vi "Rock Wall .vi"() -> ()   [LabVIEW 2015]
uses:
  AutoEnum.ctl
panel:
  in  "Encoder":dbl
  in  "Yaw":dbl
  in  "Ultrasonic":dbl
  in  "Distance Goal":dbl
  out "Rock Wall On":bool
  out "Motor Speed":dbl
  in  "Clear Error":bool
  in  "To Distance":bool
  out "Rest_Encoder":bool
  out "Rest_Gyro":bool
  in  "Enable":bool
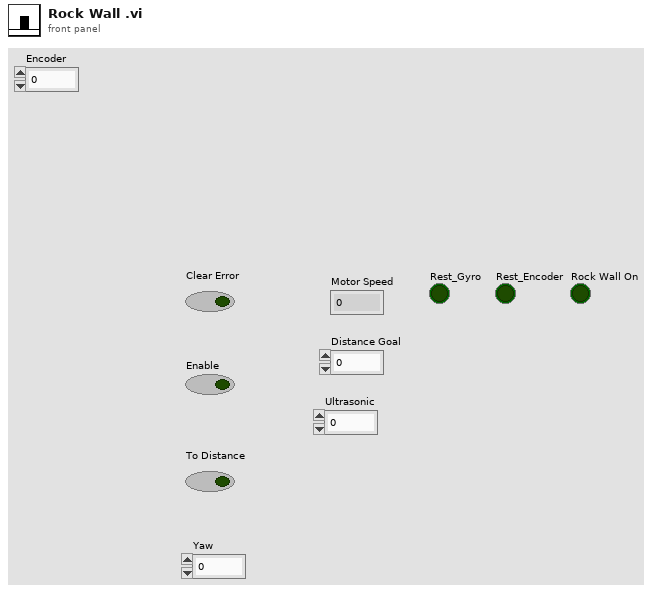
[diagram p1: front panel]
types:
  T1 = typedef "AutoEnum.ctl" = enum16{"Off", "ResetVar", "ResetOff", "BeforeTeeter", "LowerArm", "DriveForward", "Stop"}
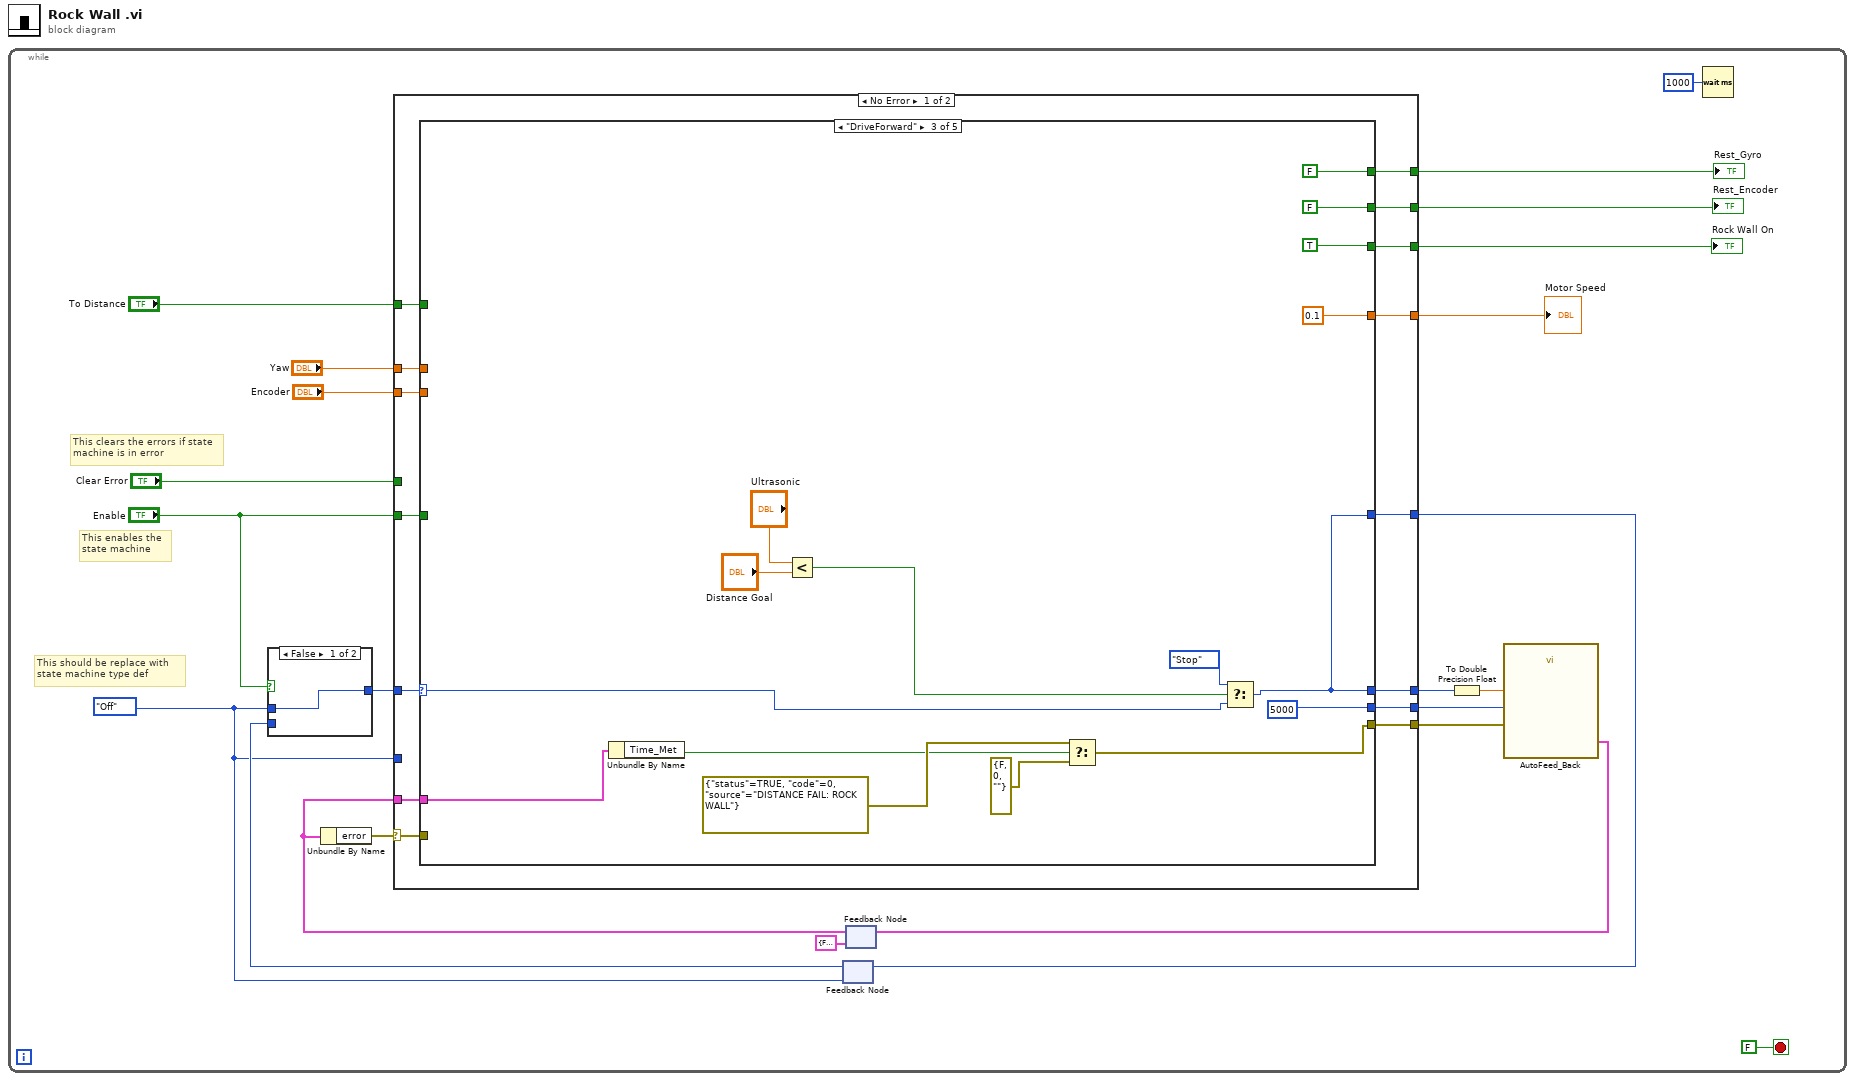
[diagram p0: block diagram]
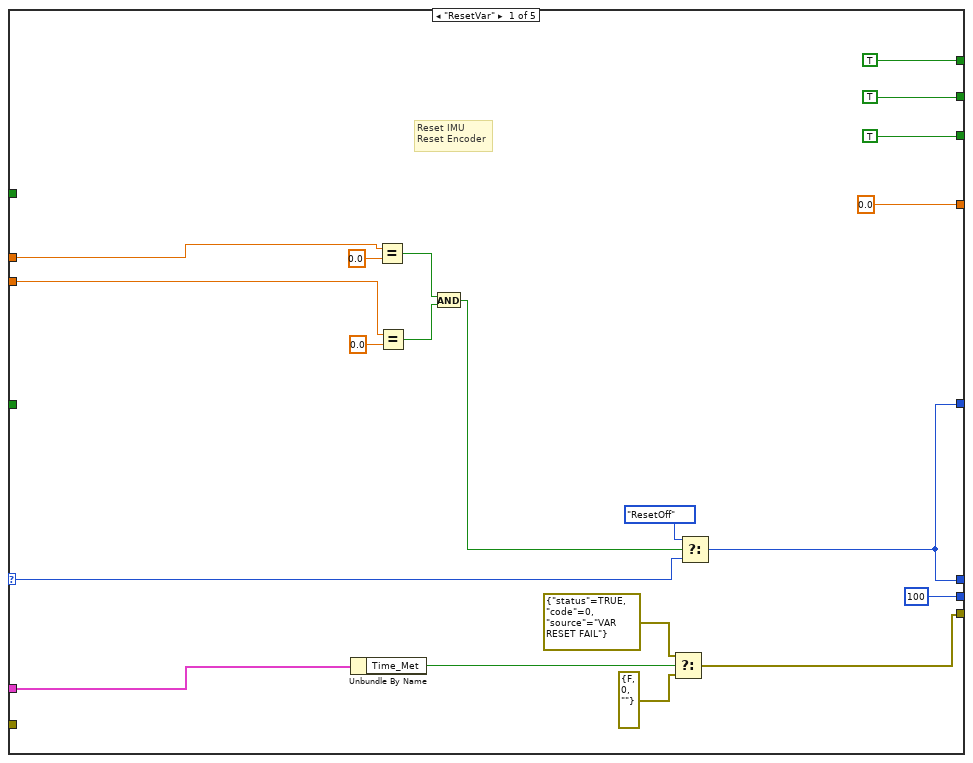
[diagram p3: hidden frame]
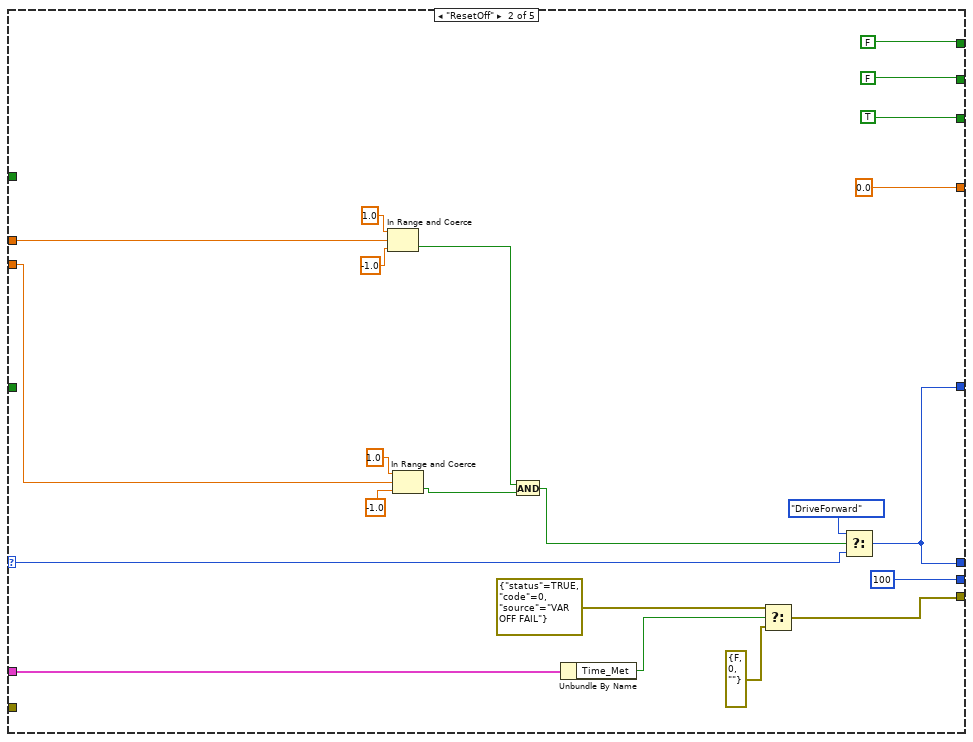
[diagram p4: hidden frame]
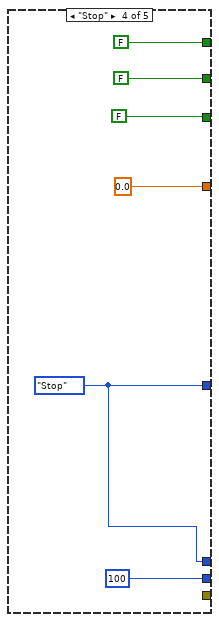
[diagram p5: hidden frame]
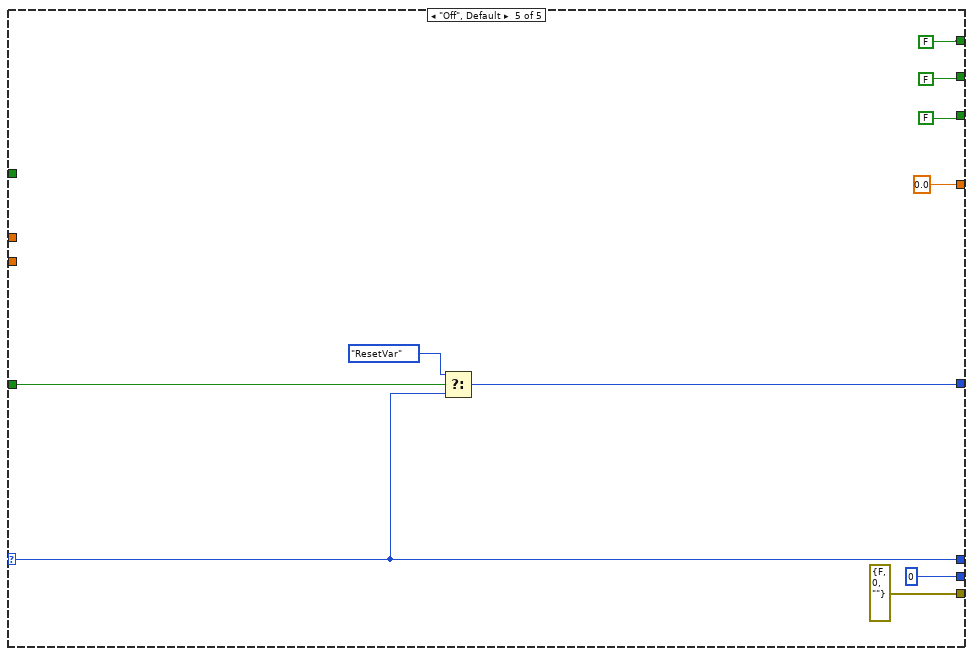
[diagram p6: hidden frame]
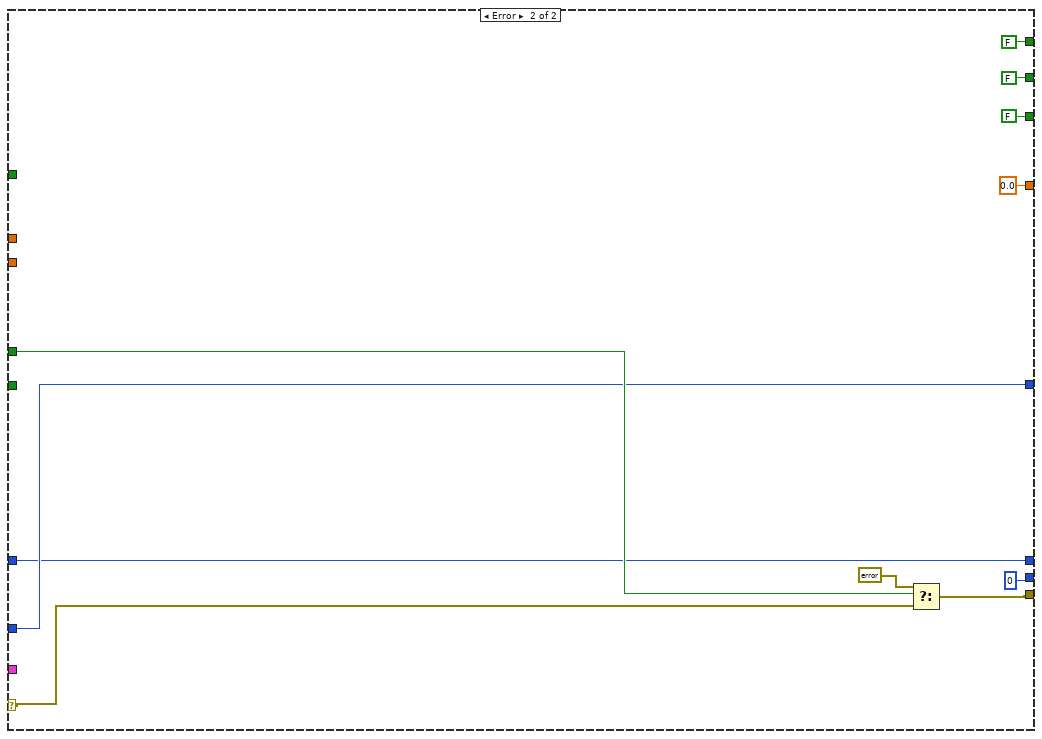
[diagram p7: hidden frame]
diagram:
  n1 = while {
    stop <- FALSE stop-if-true
    w5 = AutoEnum."Off"
    # "This clears the errors if state \nmachine is in error"
    # "This enables the \nstate machine"
    # "This should be replace with \nstate machine type def"
    n2 = feedback #1(w5) -> (w8:T1)
    n3 = case shown="False" "Enable" {
      tunnel: w5 -> [w24 _]
      tunnel: [w24 w25] -> w9
      tunnel: w8 -> [_ w25]
      frame False {
      }
      frame True {
      }
    }
    n4 = feedback #2(cluster{"Time_Met":bool, "error ":errorcluster} {"Time_Met"=FALSE, "error "={"status"=FALSE, "code"=0, "source"=""}} ("Feedback_State")) -> (w11:cluster{"Time_Met":bool, "error ":errorcluster})
    n5 = Unbundle By Name(w11) -> ("error"=w13:errorcluster)
    n6 = case shown="No Error" w13 {
      selector: w13 -> [w32 w121]
      tunnel: [w40 FALSE] -> w23
      tunnel: [w39 FALSE] -> w22
      tunnel: "To Distance" -> [w38 _]
      tunnel: [w37 w118] -> w20
      tunnel: [w36 w117] -> w7
      tunnel: [w35 0] -> w17
      tunnel: [w34 w122] -> w16
      tunnel: "Clear Error" -> [_ w120]
      tunnel: w11 -> [w33 _]
      tunnel: "Enable" -> [w31 _]
      tunnel: w9 -> [w30 w117]
      tunnel: w5 -> [_ w118]
      tunnel: [w29 0.0] -> w4
      tunnel: [w28 FALSE] -> w3
      tunnel: "Yaw" -> [w27 _]
      tunnel: "Encoder" -> [w26 _]
      frame No Error {
        n7 = case shown="\"DriveForward\"" w30 {
          selector: w30 -> [w53 w75 w90 _ w109]
          tunnel: [TRUE FALSE FALSE FALSE FALSE] -> w40
          tunnel: [TRUE FALSE FALSE FALSE FALSE] -> w39
          tunnel: [w52 w74 w91 w99 w109] -> w36
          tunnel: [100 100 5000 100 0] -> w35
          tunnel: [w52 w74 w91 w99 w108] -> w37
          tunnel: w38 -> [_ _ _ _ _]
          tunnel: [w48 w66 w83 _ errorcluster {"status"=FALSE, "code"=0, "source"=""} ("error")] -> w34
          tunnel: w33 -> [w54 w76 w94 _ _]
          tunnel: w32 -> [_ _ _ _ _]
          tunnel: w31 -> [_ _ _ _ w110]
          tunnel: [0.0 0.0 0.1 0.0 0.0] -> w29
          tunnel: [TRUE TRUE TRUE FALSE FALSE] -> w28
          tunnel: w27 -> [w46 w68 _ _ _]
          tunnel: w26 -> [w44 w67 _ _ _]
          frame "ResetVar" {
            # "Reset IMU\nReset Encoder"
            n8 = Unbundle By Name(w54) -> ("Time_Met"=w51:bool)
            n9 = Equal?(x=w46, y=0.0) -> (x = y?=w43:bool)
            n10 = Equal?(x=w44, y=0.0) -> (x = y?=w42:bool)
            n11 = And(x=w43, y=w42) -> (x .and. y?=w41:bool)
            n12 = Select(t=errorcluster {"status"=TRUE, "code"=0, "source"="VAR RESET FAIL"} ("error"), s=w51, f=errorcluster {"status"=FALSE, "code"=0, "source"=""} ("error")) -> (s? t:f=w48:errorcluster)
            n13 = Select(t=AutoEnum."ResetOff", s=w41, f=w53) -> (s? t:f=w52:T1)
          }
          frame "ResetOff" {
            n14 = In Range and Coerce(upper limit=1.0, x=w68, lower limit=-1.0) -> (In Range?=w71:bool)  [unwired: 1 out]
            n15 = In Range and Coerce(upper limit=1.0, x=w67, lower limit=-1.0) -> (In Range?=w69:bool)  [unwired: 1 out]
            n16 = And(x=w71, y=w69) -> (x .and. y?=w62:bool)
            n17 = Unbundle By Name(w76) -> ("Time_Met"=w63:bool)
            n18 = Select(t=errorcluster {"status"=TRUE, "code"=0, "source"="VAR OFF FAIL"} ("error"), s=w63, f=errorcluster {"status"=FALSE, "code"=0, "source"=""} ("error")) -> (s? t:f=w66:errorcluster)
            n19 = Select(t=AutoEnum."DriveForward", s=w62, f=w75) -> (s? t:f=w74:T1)
          }
          frame "DriveForward" {
            n20 = Unbundle By Name(w94) -> ("Time_Met"=w87:bool)
            n21 = Less?(x="Ultrasonic", y="Distance Goal") -> (x < y?=w84:bool)
            n22 = Select(t=errorcluster {"status"=TRUE, "code"=0, "source"="DISTANCE FAIL: ROCK WALL"} ("error"), s=w87, f=errorcluster {"status"=FALSE, "code"=0, "source"=""} ("error")) -> (s? t:f=w83:errorcluster)
            n23 = Select(t=AutoEnum."Stop", s=w84, f=w90) -> (s? t:f=w91:T1)
          }
          frame "Stop" {
            w99 = AutoEnum."Stop"
          }
          frame "Off", Default {
            n24 = Select(t=AutoEnum."ResetVar", s=w110, f=w109) -> (s? t:f=w108:T1)
          }
        }
      }
      frame Error {
        n25 = Select(t=errorcluster {"status"=FALSE, "code"=0, "source"=""}, s=w120, f=w121) -> (s? t:f=w122:errorcluster)
      }
    }
    "Rest_Gyro" <- w23
    "Rest_Encoder" <- w22
    "Motor Speed" <- w4
    "Rock Wall On" <- w3
    n26 = feedback-in #1(w20) -> ()
    n27 = To Double Precision Float(number=w7) -> (double precision float=w6:dbl)
    n28 = call "AutoFeed_Back.vi"("error"=w16, "Time (ms)"=w17, "State"=w6) -> ("Feedback_State"=w15:cluster{"Time_Met":bool, "error ":errorcluster})  [unwired: 8 in]
    n29 = feedback-in #2(w15) -> ()
    n30 = Wait (ms)(milliseconds to wait=u32 1000) -> ()  [unwired: 1 out]
  }
